vi "Multiply_IQ_subtract.vi"(6 "Sin":fxp<+/-,16,0>, 7 "Cos":fxp<+/-,16,0>, 8 "input valid":bool=TRUE, 10 "Q":fxp<+/-,16,14>, 11 "I":fxp<+/-,16,14>) -> (0 "output valid":bool, 3 "Z":i16)   [LabVIEW 2013]
doc: "Calculates\nI*Cos(wt)-Q*Sin(wt)"
uses:
  <vilib>/rvi/FXPMathLib/FxpConvert/subVIs/nifxpmath_Convert_SimConfig.ctl
  <vilib>/fxp/LVFixedPointQuantizationPolicyTypeDef.ctl
  <vilib>/fxp/LVFixedPointOverflowPolicyTypeDef.ctl
  <vilib>/rvi/FXPMathLib/FxpConvert/simVIs/DllFxpConvertTemp_sub.vi
  <vilib>/rvi/FXPMathLib/FxpInterpret/XNode/nifxpmath_Interpret.xnode
  <vilib>/rvi/FXPMathLib/FxpConvert/XNode/nifxpmath_Convert.xnode
  <vilib>/rvi/FXPMathLib/FxpSub/XNode/nifxpmath_Sub.xnode
  <vilib>/rvi/FXPMathLib/FxpMul/XNode/nifxpmath_Multiplier.xnode
  <vilib>/rvi/FXPMathLib/sim/FxpSim.dll
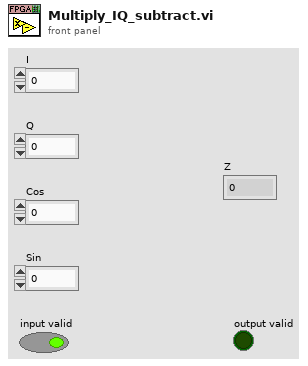
[diagram p1: front panel]
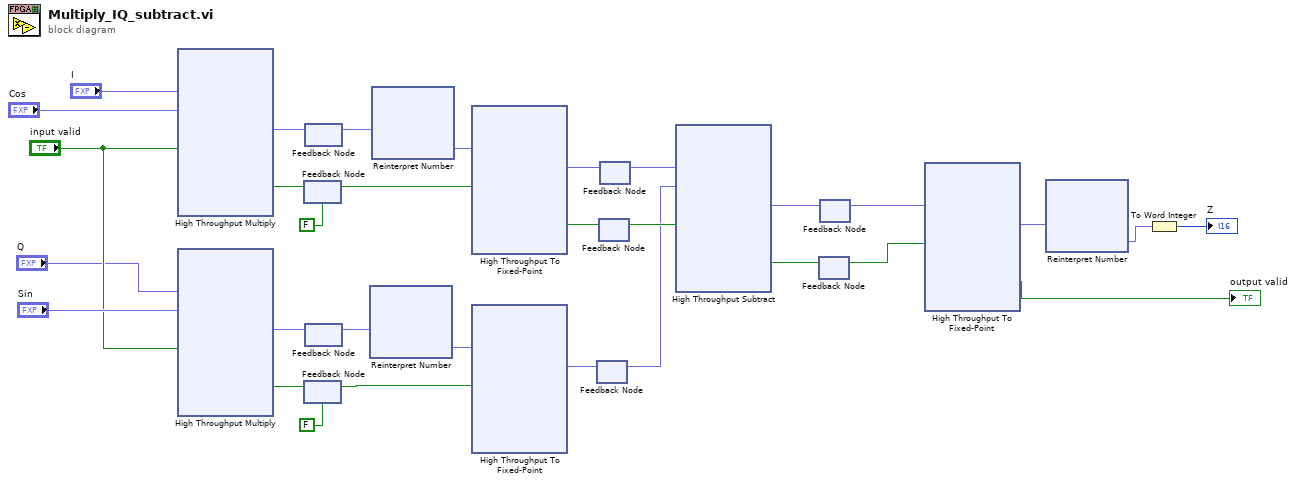
[diagram p0: block diagram]
diagram:
  n1 = xnode ("High Throughput Multiply")("x"="I", "y"="Cos", "input valid"="input valid") -> ("x*y"=w31:fxp<+/-,32,14>, "output valid"=w30:bool)  [unwired: 1 in, 1 out]
  n2 = xnode ("High Throughput Multiply")("x"="Q", "y"="Sin", "input valid"="input valid") -> ("x*y"=w21:fxp<+/-,32,14>, "output valid"=w20:bool)  [unwired: 1 in, 1 out]
  n3 = feedback #1(FALSE ("output valid")) -> (w24:bool)
  n4 = feedback-in #1(w30) -> ()
  n5 = feedback #2(FALSE ("output valid")) -> (w23:bool)
  n6 = feedback-in #2(w20) -> ()
  n7 = feedback #3() -> (w4:fxp<+/-,32,14>)  [unwired: 1 in]
  n8 = feedback-in #3(w31) -> ()
  n9 = feedback #4() -> (w6:fxp<+/-,32,14>)  [unwired: 1 in]
  n10 = feedback-in #4(w21) -> ()
  n11 = xnode "Reinterpret Number"("x"=w6) -> ("y"=w5:fxp<+/-,32,16>)
  n12 = xnode "Reinterpret Number"("x"=w4) -> ("y"=w3:fxp<+/-,32,16>)
  n13 = xnode "High Throughput To Fixed-Point"("x"=w3, "input valid"=w24) -> ("y"=w12:fxp<+/-,16,14>, "output valid"=w11:bool)  [unwired: 1 in, 1 out]
  n14 = xnode "High Throughput To Fixed-Point"("x"=w5, "input valid"=w23) -> ("y"=w9:fxp<+/-,16,14>)  [unwired: 1 in, 2 out]
  n15 = feedback #5() -> (w8:fxp<+/-,16,14>)  [unwired: 1 in]
  n16 = feedback-in #5(w9) -> ()
  n17 = feedback #6() -> (w10:bool)  [unwired: 1 in]
  n18 = feedback-in #6(w11) -> ()
  n19 = feedback #7() -> (w7:fxp<+/-,16,14>)  [unwired: 1 in]
  n20 = feedback-in #7(w12) -> ()
  n21 = xnode "High Throughput Subtract"("x"=w7, "y"=w8, "input valid"=w10) -> ("x-y"=w19:fxp<+/-,17,15>, "output valid"=w17:bool)  [unwired: 1 in, 1 out]
  n22 = feedback #8() -> (w16:bool)  [unwired: 1 in]
  n23 = feedback-in #8(w17) -> ()
  n24 = feedback #9() -> (w18:fxp<+/-,17,15>)  [unwired: 1 in]
  n25 = feedback-in #9(w19) -> ()
  n26 = xnode "High Throughput To Fixed-Point"("x"=w18, "input valid"=w16) -> ("y"=w2:fxp<+/-,16,14>, "output valid"=→"output valid":bool)  [unwired: 1 in, 1 out]
  n27 = xnode "Reinterpret Number"("x"=w2) -> ("y"=w1:fxp<+/-,16,16>)
  n28 = To Word Integer(number=w1) -> (16bit integer=→"Z":i16)
